vi "DriveAndWiggle.vi"(7 "Wiggle amount":dbl, 8 "error in":errorcluster, 9 "Wiggle Period (ms)":u32, 10 "Time (ms)":u32, 11 "Speed/Direction":dbl) -> (0 "error out":errorcluster)   [LabVIEW 2016]
doc: "Drives forward while wiggling"
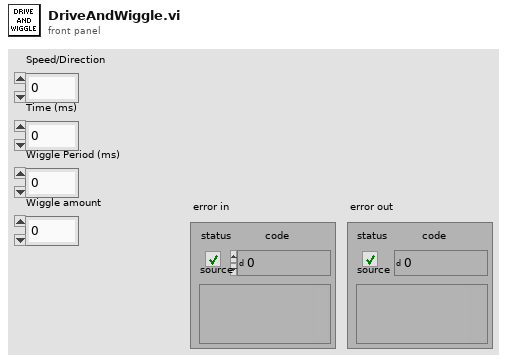
[diagram p1: front panel]
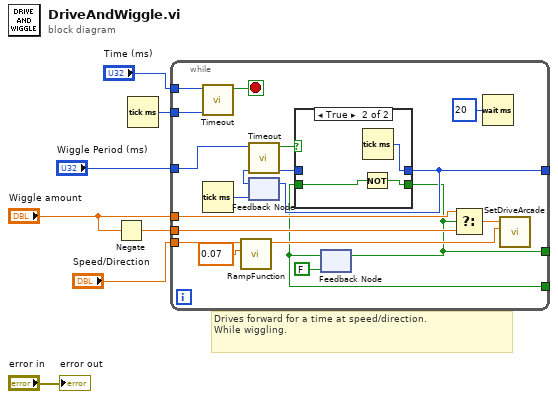
[diagram p0: block diagram]
diagram:
  # "Drives forward for a time at speed/direction.\nWhile wiggling."
  n1 = Negate(x="Wiggle amount") -> (-x=w1:dbl)
  n2 = Tick Count (ms)() -> (millisecond timer value=w5:u32)
  n3 = while {
    tunnel: "Time (ms)" -> [w26]
    tunnel: "Speed/Direction" -> [w22]
    tunnel: w5 -> [w24]
    tunnel: "Wiggle Period (ms)" -> [w20]
    tunnel: "Wiggle amount" -> [w19]
    tunnel: w1 -> [w18]
    tunnel: [w10] -> _
    tunnel: [w11] -> _
    tunnel: [w13] -> _
    stop <- w25 stop-if-true
    n4 = call "Timeout.vi"("Start Time In"=w24, "Time Limit (ms)"=w26) -> ("Timeout"=w25:bool)  [unwired: 8 in, 1 out]
    n5 = Tick Count (ms)() -> (millisecond timer value=w14:u32)
    n6 = call "RampFunction.vi"("Max Rate"=0.07, "Input"=w22) -> ("Output"=w21:dbl)  [unwired: 9 in]
    n7 = feedback #1(w14) -> (w12:u32)
    n8 = call "Timeout.vi"("Start Time In"=w12, "Time Limit (ms)"=w20) -> ("Start Time Out"=w15:u32, "Timeout"=w16:bool)  [unwired: 8 in]
    n9 = feedback #2(FALSE) -> (w10:bool)
    n10 = case shown="True" w16 {
      tunnel: w10 -> [w28 w31]
      tunnel: [w28 w30] -> w11
      tunnel: w15 -> [w27 _]
      tunnel: [w27 w29] -> w13
      frame False {
      }
      frame True {
        n11 = Not(x=w31) -> (.not. x?=w30:bool)
        n12 = Tick Count (ms)() -> (millisecond timer value=w29:u32)
      }
    }
    n13 = feedback-in #1(w13) -> ()
    n14 = feedback-in #2(w11) -> ()
    n15 = Select(t=w19, s=w11, f=w18) -> (s? t:f=w17:dbl)
    n16 = Wait (ms)(milliseconds to wait=u32 20) -> ()  [unwired: 1 out]
    n17 = call "SetDriveArcade.vi"("Forward"=w21, "Turn"=w17) -> ()  [unwired: 9 in, 1 out]
  }
  "error out" <- "error in"
